vi "Query Modulation Mode.vi"(8 "error in (no error)":errorcluster, 10 "Channel (0: Channel 1)":T1 items=["Channel 1", "Channel 2"], 11 "VISA resource name":refnum<visa-resource-name>) -> (0 "error out":errorcluster, 2 "Modulation Mode":u16(ring) items=["Not In Modulation Mode", "AM", "FM", "PM", "FSK", "PWM"], 3 "VISA resource name out":refnum<visa-resource-name>)   [LabVIEW 2017, in "Tektronix AFG 3000 Series.lvlib"]
uses:
  Tektronix AFG 3000 Series.lvlib
  controls.llb/Channel.ctl
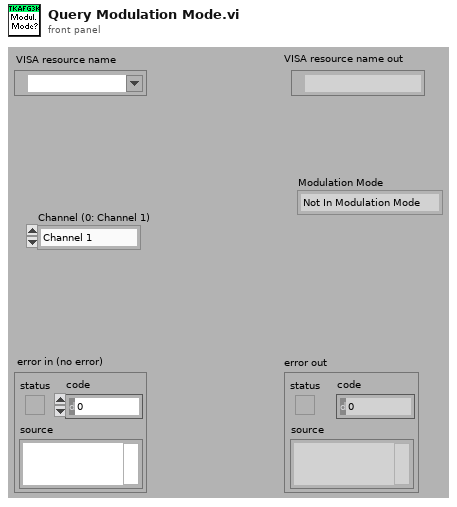
[diagram p1: front panel]
types:
  T1 = typedef "Channel.ctl" = u16
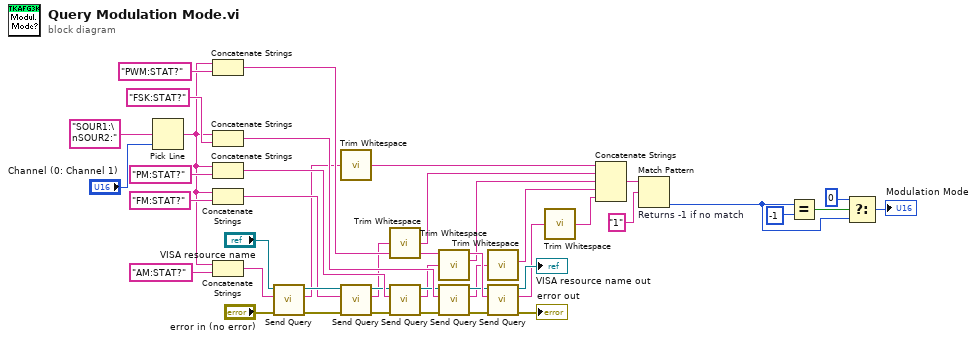
[diagram p0: block diagram]
diagram:
  n1 = Pick Line(multi-line string="SOUR1:\nSOUR2:" ("string (\"\")"), line index="Channel (0: Channel 1)") -> (output string=w16:string)  [unwired: 1 out]
  n2 = Concatenate Strings(w16, "PWM:STAT?" ("format string")) -> (w15:string)
  n3 = Concatenate Strings(w16, "FSK:STAT?" ("format string")) -> (w27:string)
  n4 = Concatenate Strings(w16, "PM:STAT?" ("format string")) -> (w31:string)
  n5 = Concatenate Strings(w16, "FM:STAT?" ("format string")) -> (w34:string)
  n6 = Concatenate Strings(w16, "AM:STAT?" ("format string")) -> (w38:string)
  n7 = call "Send Query.vi"("error in (no error)"="error in (no error)", "write buffer"=w38, "VISA resource name"="VISA resource name") -> ("error out"=w33:errorcluster, "read buffer"=w2:string, "VISA resource name out"=w35:refnum<visa-resource-name>)  [unwired: 1 in, 5 out]
  n8 = call <vilib>:"Trim Whitespace.vi"("string"=w2) -> ("trimmed string"=w1:string)  [unwired: 1 in]
  n9 = call "Send Query.vi"("error in (no error)"=w33, "write buffer"=w34, "VISA resource name"=w35) -> ("error out"=w29:errorcluster, "read buffer"=w3:string, "VISA resource name out"=w30:refnum<visa-resource-name>)  [unwired: 1 in, 5 out]
  n10 = call <vilib>:"Trim Whitespace.vi"("string"=w3) -> ("trimmed string"=w4:string)  [unwired: 1 in]
  n11 = call "Send Query.vi"("error in (no error)"=w29, "write buffer"=w31, "VISA resource name"=w30) -> ("error out"=w25:errorcluster, "read buffer"=w6:string, "VISA resource name out"=w26:refnum<visa-resource-name>)  [unwired: 1 in, 5 out]
  n12 = call <vilib>:"Trim Whitespace.vi"("string"=w6) -> ("trimmed string"=w5:string)  [unwired: 1 in]
  n13 = call "Send Query.vi"("error in (no error)"=w25, "write buffer"=w27, "VISA resource name"=w26) -> ("error out"=w12:errorcluster, "read buffer"=w10:string, "VISA resource name out"=w14:refnum<visa-resource-name>)  [unwired: 1 in, 5 out]
  n14 = call <vilib>:"Trim Whitespace.vi"("string"=w10) -> ("trimmed string"=w9:string)  [unwired: 1 in]
  n15 = call "Send Query.vi"("error in (no error)"=w12, "write buffer"=w15, "VISA resource name"=w14) -> ("error out"=→"error out":errorcluster, "read buffer"=w8:string, "VISA resource name out"=→"VISA resource name out":refnum<visa-resource-name>)  [unwired: 1 in, 5 out]
  n16 = call <vilib>:"Trim Whitespace.vi"("string"=w8) -> ("trimmed string"=w7:string)  [unwired: 1 in]
  n17 = Concatenate Strings(w1, w4, w5, w9, w7) -> (w23:string)
  n18 = Match Pattern "Returns -1 if no match"(string=w23, regular expression="1") -> (offset past match=w19:i32)  [unwired: 4 out]
  n19 = Equal?(x=w19, y=-1) -> (x = y?=w21:bool)
  n20 = Select(t=0, s=w21, f=w19) -> (s? t:f=→"Modulation Mode":i32)
